vi "API.vi"() -> (1 "Names":string[](array[string]), 2 "Help Directory":path=path "Z:/Windows Common/JSONtext", 3 "API":path[](array[path]))   [LabVIEW 2017]
uses:
  <userlib>/_OpenG.lib/file/file.llb/Strip Path Extension - String__ogtk.vi
panel:
  in  "Starting Path":path=path "C:/git/JSONtext/Array of Variants to JSON Array.vi"
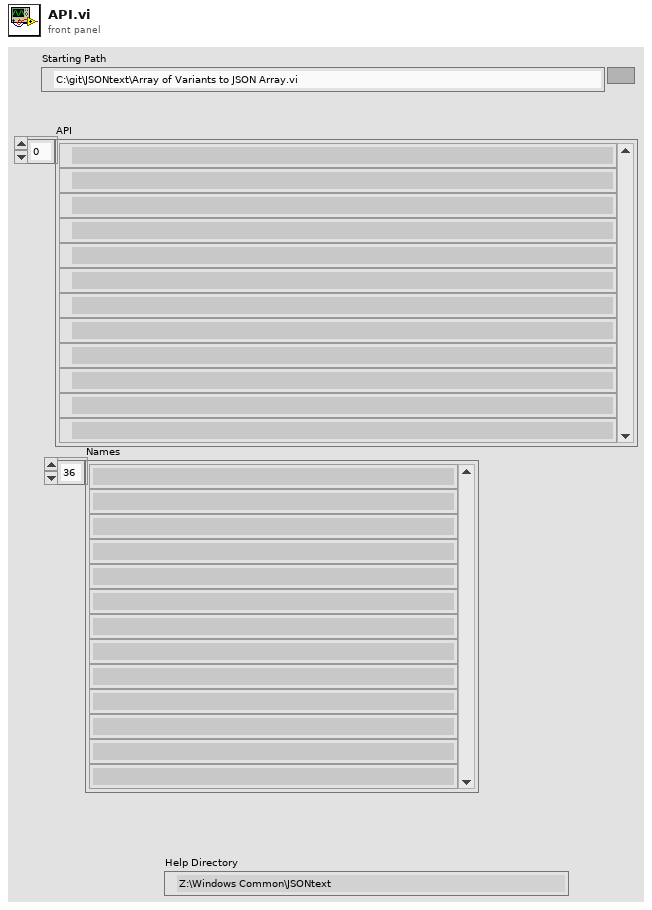
[diagram p1: front panel]
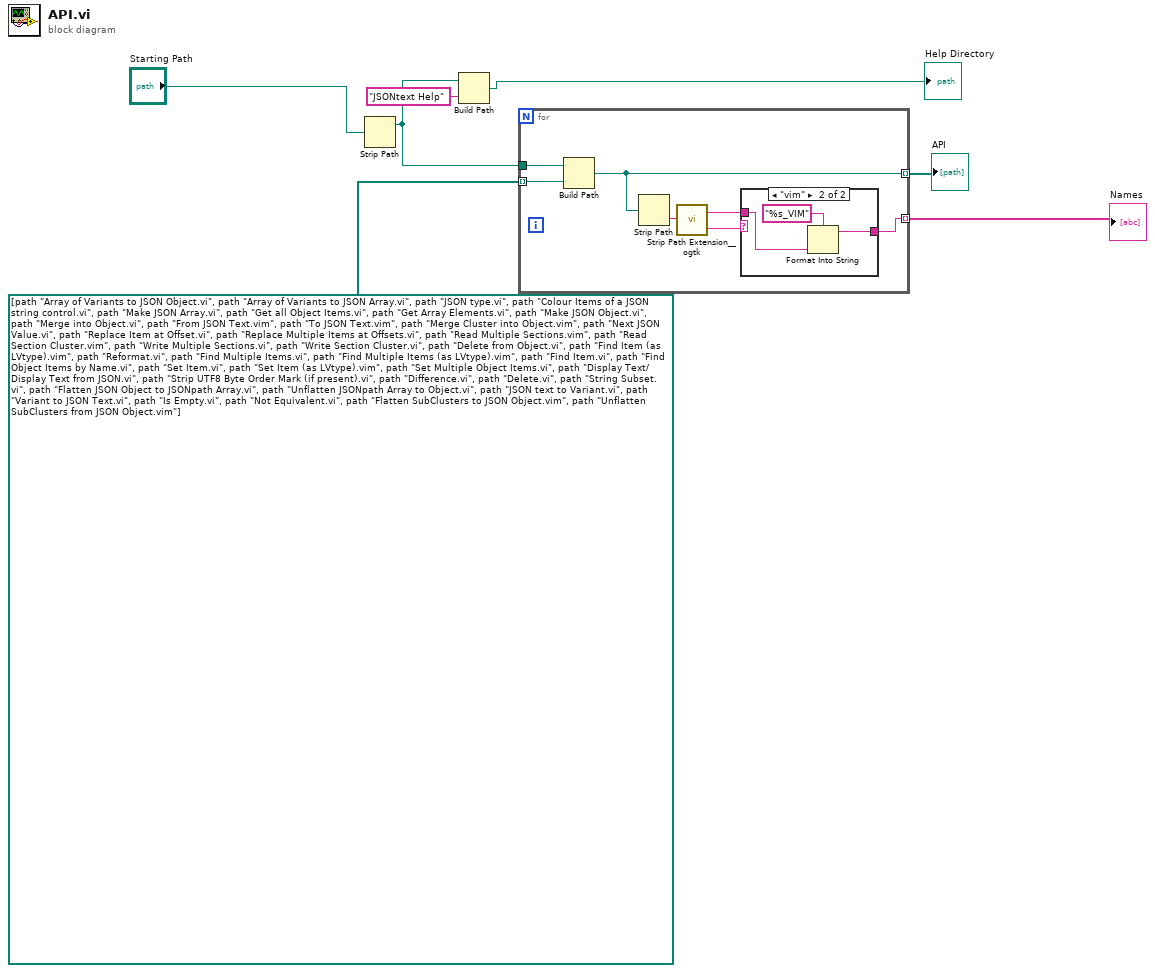
[diagram p0: block diagram]
diagram:
  n1 = Strip Path(path="Starting Path") -> (stripped path=w4:path)  [unwired: 1 out]
  n2 = Build Path(base path=w4, name or relative path="JSONtext Help") -> (appended path=→"Help Directory":path)
  n3 = for {
    tunnel: w4 -> [w14]
    tunnel: path[] [path "Array of Variants to JSON Object.vi", path "Array of Variants to JSON Array.vi", path "JSON type.vi", path "Colour Items of a JSON string control.vi", path "Make JSON Array.vi", path "Get all Object Items.vi", path "Get Array Elements.vi", path "Make JSON Object.vi", path "Merge into Object.vi", path "From JSON Text.vim", path "To JSON Text.vim", path "Merge Cluster into Object.vim", path "Next JSON Value.vi", path "Replace Item at Offset.vi", path "Replace Multiple Items at Offsets.vi", path "Read Multiple Sections.vim", path "Read Section Cluster.vim", path "Write Multiple Sections.vi", path "Write Section Cluster.vi", path "Delete from Object.vi", path "Find Item (as LVtype).vim", path "Reformat.vi", path "Find Multiple Items.vi", path "Find Multiple Items (as LVtype).vim", path "Find Item.vi", path "Find Object Items by Name.vi", path "Set Item.vi", path "Set Item (as LVtype).vim", path "Set Multiple Object Items.vi", path "Display Text/Display Text from JSON.vi", path "Strip UTF8 Byte Order Mark (if present).vi", path "Difference.vi", path "Delete.vi", path "String Subset.vi", path "Flatten JSON Object to JSONpath Array.vi", path "Unflatten JSONpath Array to Object.vi", path "JSON text to Variant.vi", path "Variant to JSON Text.vi", path "Is Empty.vi", path "Not Equivalent.vi", path "Flatten SubClusters to JSON Object.vim", path "Unflatten SubClusters from JSON Object.vim"] -> [w13] mode=indexing
    tunnel: [w12] -> w5 mode=indexing
    tunnel: [w8] -> w1 mode=indexing
    n4 = Build Path(base path=w14, name or relative path=w13) -> (appended path=w12:path)
    n5 = Strip Path(path=w12) -> (name=w11:string)  [unwired: 1 out]
    n6 = call-poly <userlib>:"Strip Path Extension__ogtk.vi"("path"=w11) -> ("root"=w9:string, "extension"=w10:string)
    n7 = case shown="\"vim\"" w10 {
      tunnel: w9 -> [w15 w18]
      tunnel: [w15 w17] -> w8
      frame Default {
      }
      frame "vim" {
        n8 = Format Into String(format string="%s_VIM", w18) -> (resulting string=w17:string)  [unwired: 2 in, 1 out]
      }
    }
  }
  "API" <- w5
  "Names" <- w1
